vi "Signal_type.vi"(8 "error in (no error)":errorcluster, 10 "Tipo de señal":enum16{"Senoidal", "Cuadrada", "Triangular"}(ring), 11 "GUI_Actor in":refnum<class "GUI_Actor.lvclass">) -> (0 "error out":errorcluster, 3 "GUI_Actor out":refnum<class "GUI_Actor.lvclass">)   [LabVIEW 2019, in "GUI_Actor.lvlib" / "GUI_Actor.lvclass"]
uses:
  GUI_Actor.lvclass
  GUI_Actor.lvclass/GUI_Actor.ctl
  Signal_Gen/Signal_Gen Messages/signal_type Msg/signal_type Msg.lvclass/signal_type Msg.ctl
  <vilib>/ActorFramework/Message Enqueuer/Message Enqueuer.lvclass/Message Enqueuer.ctl
  <vilib>/ActorFramework/Message Enqueuer/Enqueue.vi
  Signal_Gen/Signal_Gen Messages/signal_type Msg/signal_type Msg.lvclass
  C:/Program Files/National Instruments/LabVIEW 2019/vi.lib/ActorFramework/Message/Message.lvclass
  <vilib>/ActorFramework/Message Priority Queue/Priority Enqueue.vi
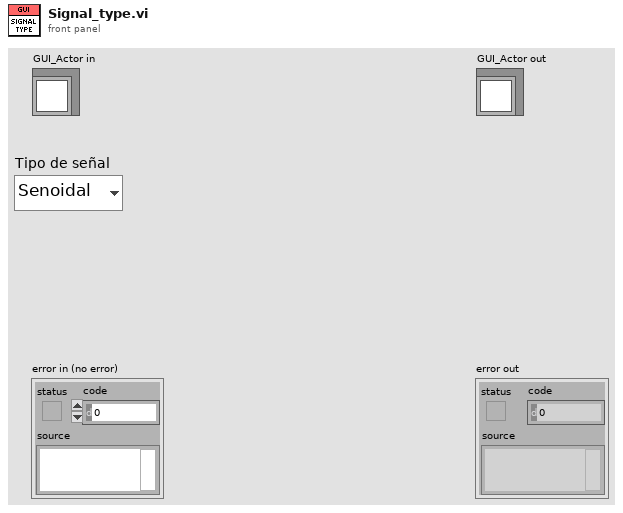
[diagram p1: front panel]
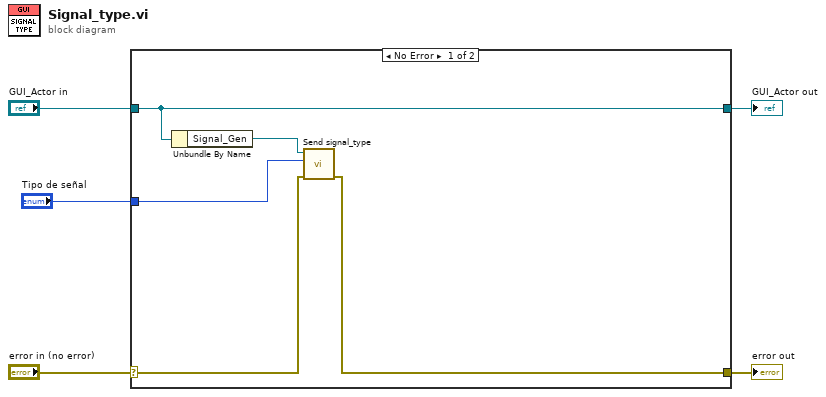
[diagram p0: block diagram]
diagram:
  n1 = case shown="No Error" "error in (no error)" {
    selector: "error in (no error)" -> [w7 w12]
    tunnel: [w6 w12] -> w4
    tunnel: [w10 w11] -> w2
    tunnel: "GUI_Actor in" -> [w10 w11]
    tunnel: "Tipo de señal" -> [w8 _]
    frame No Error {
      n2 = Unbundle By Name(w10) -> ("Signal_Gen"=w9:refnum<class "Message Enqueuer.lvclass">)
      n3 = call "Send signal_type.vi"("error in (no error)"=w7, "Tipo de señal"=w8, "Message Enqueuer"=w9) -> ("error out"=w6:errorcluster)  [unwired: 7 in, 1 out]
    }
    frame Error {
    }
  }
  "error out" <- w4
  "GUI_Actor out" <- w2
